vi "Handle getAll.vi"(8 "error in (no error)":errorcluster, 11 "Inst.MOTOR in":refnum<class "Inst.MOTOR.lvclass">) -> (0 "error out":errorcluster, 2 "getAll":variant, 3 "Inst.MOTOR out":refnum<class "Inst.MOTOR.lvclass">)   [LabVIEW 2019, in "Inst.MOTOR.lvclass"]
uses:
  Inst.MOTOR.lvclass
  Typedefs/Inst.MOTOR.getAll--Cluster.ctl
  Inst.MOTOR.lvclass/Inst.MOTOR.ctl
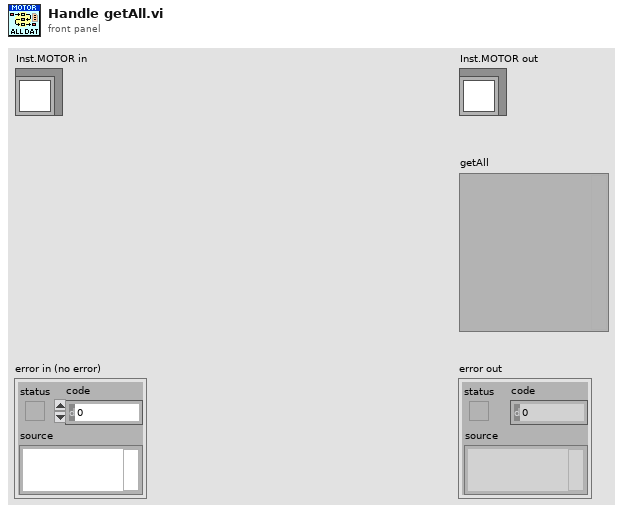
[diagram p1: front panel]
types:
  T1 = typedef "Inst.MOTOR.lvclass/Inst.MOTOR.getAll--Cluster.ctl" = cluster{"Response":string, "Forward":bool, "Stop Motor":bool, "Encoder Position":string}
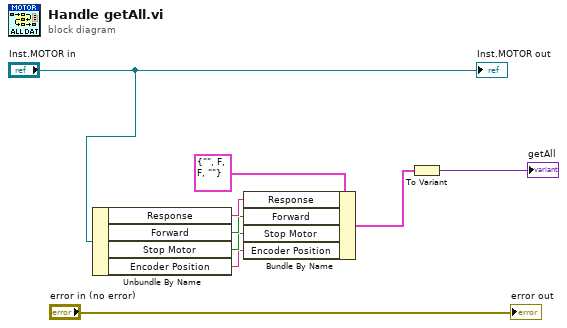
[diagram p0: block diagram]
diagram:
  n1 = Unbundle By Name("Inst.MOTOR in") -> ("Response"=w7:string, "Forward"=w6:bool, "Stop Motor"=w5:bool, "Encoder Position"=w4:string)
  n2 = Bundle By Name(cluster=T1 {"Response"="", "Forward"=FALSE, "Stop Motor"=FALSE, "Encoder Position"=""} ("getAll"), "Response"=w7, "Forward"=w6, "Stop Motor"=w5, "Encoder Position"=w4) -> (w3:T1)
  n3 = To Variant(anything=w3) -> (Variant=→"getAll":variant)
  "error out" <- "error in (no error)"
  "Inst.MOTOR out" <- "Inst.MOTOR in"
